vi "APS set point table.vi"(8 "error in (no error)":errorcluster caption="错误输入（无错误）", 9 "Point":T1, 10 "Index":i32, 11 "Axis_ID":i32) -> (0 "error out":errorcluster caption="错误输出", 1 "Point out":T1, 3 "function return":i32)   [LabVIEW 2011, in "APS168.lvlib"]
doc: "I32 FNTYPE APS_set_point_table( I32 Axis_ID, I32 Index, POINT_DATA *Point );"
uses:
  APS168.lvlib
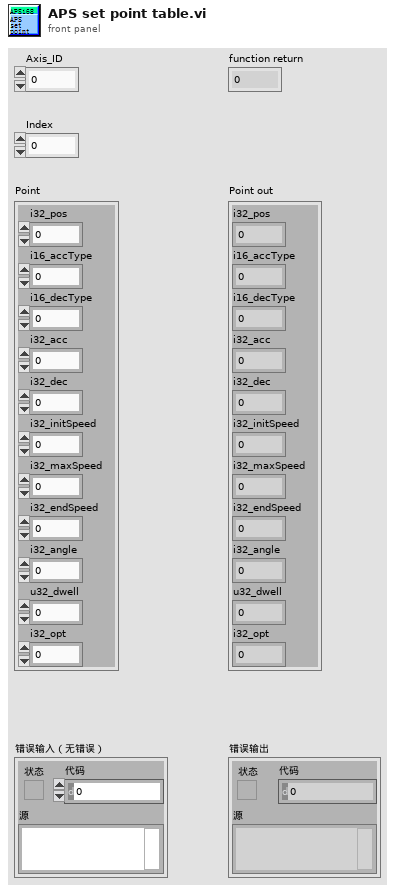
[diagram p1: front panel]
types:
  T1 = cluster{"i32_pos":i32, "i16_accType":i16, "i16_decType":i16, "i32_acc":i32, "i32_dec":i32, "i32_initSpeed":i32, "i32_maxSpeed":i32, "i32_endSpeed":i32, "i32_angle":i32, "u32_dwell":u32, "i32_opt":i32}
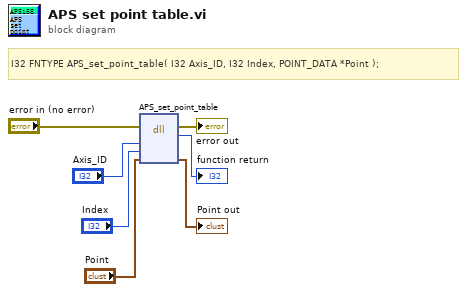
[diagram p0: block diagram]
diagram:
  # "I32 FNTYPE APS_set_point_table( I32 Axis_ID, I32 Index, POINT_DATA *Point );"
  n1 = dll-call lib="PTH1Labs E软件ADLINK 204CAPS_1_7_1_LIB line 连续运动204APS168.*" fn="APS_set_point_table"(error in="error in (no error)", "Axis_ID"="Axis_ID", "Index"="Index", "Point"="Point") -> (error out=→"error out":errorcluster, →"function return":i32, "Point"=→"Point out":T1)  [unwired: 4 in, 1 out]
